vi "FRCts20_Backend_SetDates.vi"(8 "error in (no error)":errorcluster, 11 "Time Stamp":timestamp) -> (0 "error out":errorcluster, 2 "Status":string)   [LabVIEW 2014, in "FRCts20_Backend_WebMethods.lvlib"]
uses:
  FRCts20_Backend_WebMethods.lvlib
  FRCts20_Backend_Engine.lvlib
  FRCts20_Backend_FGVOperation.ctl
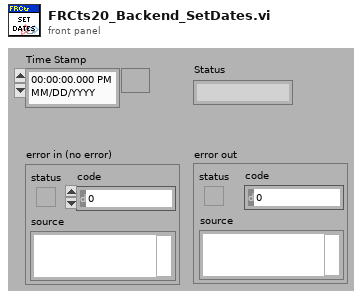
[diagram p1: front panel]
types:
  T1 = typedef "FRCts20_Backend_Engine.lvlib/FRCts20_Backend_FGVOperation.ctl" = enum16{"Initialize", "EnqueueMessage", "EnqueueDataReturn", "FlushMessage", "FlushDataReturn"}
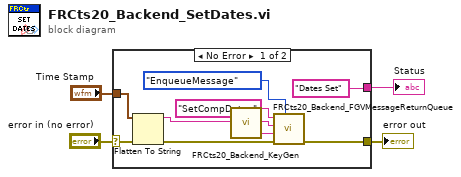
[diagram p0: block diagram]
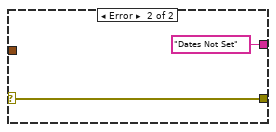
[diagram p2: hidden frame]
diagram:
  n1 = case shown="No Error" "error in (no error)" {
    selector: "error in (no error)" -> [w11 w15]
    tunnel: "Time Stamp" -> [w13 _]
    tunnel: [w6 w15] -> w2
    tunnel: ["Dates Set" "Dates Not Set"] -> w1
    frame No Error {
      n2 = Flatten To String(anything=w13, error in (no error)=w11) -> (data string=w12:string, error out=w10:errorcluster)  [unwired: 2 in, 1 out]
      n3 = call "FRCts20_Backend_KeyGen.vi"() -> ("Keygen"=w9:string)  [unwired: 27 in]
      n4 = call "FRCts20_Backend_FGVMessageReturnQueue.vi"("Operation"=FRCts20_Backend_FGVOperation."EnqueueMessage", "error in (no error)"=w10, "Key"=w9, "Message Value"=w12, "Message Name"="SetCompDates") -> ("error out"=w6:errorcluster)  [unwired: 3 in, 1 out]
    }
    frame Error {
    }
  }
  "error out" <- w2
  "Status" <- w1
